vi "Smart Relay Test.vi"(8 "error in":errorcluster, 11 "IED Test in":refnum<class "IED Test.lvclass">) -> (0 "error out":errorcluster, 2 "Test Result":T1=enum."Success", 3 "IED Test out":refnum<class "IED Test.lvclass">)   [LabVIEW 2018, in "IED Test Framework.lvlib" / "IED Test.lvclass"]
uses:
  IED Test.lvclass
  C:/Program Files (x86)/National Instruments/LabVIEW 2018/vi.lib/ActorFramework/Actor/Actor.lvclass
  C:/Users/Administrator/Desktop/2018LabVIEW EMS/EMS Generic Actor/EMS Generic/EMS Generic.lvclass
  Controls/Test Result.ctl
  <vilib>/ORNL/CSEISMIC DDS/CSEISMIC DDS Base/Data Types/Controls/DeviceClass Selector.ctl
  Smart Relay Actor/Smart Relay/Smart Relay.lvclass
  C:/Users/Administrator/Desktop/2018LabVIEW EMS/IED Actors/Device DDS Communications Framework/Device DDS Communications/Device DDS Communications.lvclass
  <vilib>/ORNL/CSEISMIC DDS/CSEISMIC DDS Base/CSEISMIC DDS.lvclass/CSEISMIC DDS.ctl
  <vilib>/ORNL/CSEISMIC DDS/CSEISMIC DDS Base/Data Types/Controls/DeviceID.ctl
  <vilib>/ActorFramework/Message Enqueuer/Message Enqueuer.lvclass/Message Enqueuer.ctl
  <vilib>/ORNL/CSEISMIC DDS/CSEISMIC DDS Base/Accessors/Write DDS Reference.vi
  <vilib>/ORNL/CSEISMIC DDS/CSEISMIC DDS Base/Accessors/Read DDS Reference.vi
  <vilib>/ActorFramework/Message Enqueuer/Enqueue.vi
  <vilib>/ORNL/CSEISMIC DDS/DDS Writer/DDS Writer.lvclass
  C:/Program Files (x86)/National Instruments/LabVIEW 2018/vi.lib/ORNL/CSEISMIC DDS/CSEISMIC DDS Base/CSEISMIC DDS.lvclass
  <vilib>/ActorFramework/Stop Msg/Stop Msg.lvclass
  C:/Program Files (x86)/National Instruments/LabVIEW 2018/vi.lib/ActorFramework/Message/Message.lvclass
  <vilib>/ORNL/CSEISMIC DDS/CSEISMIC DDS Base/Error Handler.vi
  <vilib>/ActorFramework/Message Priority Queue/Priority Enqueue.vi
  <vilib>/ORNL/CSEISMIC DDS/CSEISMIC DDS Base/CSEISMIC DDS.lvclass
  Device DDS Communications Framework/Device DDS Communications/Device DDS Communications.lvclass
  <vilib>/ActorFramework/Actor/Actor.lvclass
  EMS Generic Actor/EMS Generic/EMS Generic.lvclass
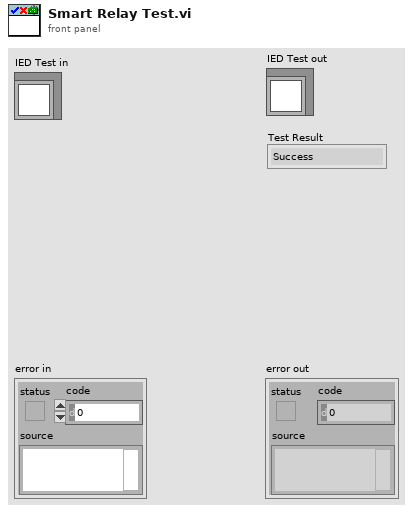
[diagram p1: front panel]
types:
  T1 = typedef "IED Test Framework.lvlib/IED Test.lvclass/Test Result.ctl" = enum16{"Invalid", "Success", "Failure", "Error", "Timeout"}
  T2 = typedef "CSEISMIC DDS.lvlib/CSEISMIC DDS.lvclass/DeviceID.ctl" = string
  T3 = typedef "CSEISMIC DDS.lvlib/CSEISMIC DDS.lvclass/DeviceClass Selector.ctl" = u16
  T4 = typedef "CSEISMIC DDS.lvlib/CSEISMIC DDS.lvclass/SmartRelay_Info.ctl" = cluster{"DeviceID":T2, "LineConfig":u8[], "NominalVoltage(V)":dbl}
  T5 = typedef "CSEISMIC DDS.lvlib/CSEISMIC DDS.lvclass/SmartRelay_Measurement.ctl" = cluster{"DeviceID":T2, "PrimaryVoltage":dbl[], "SecondaryVoltage":dbl[], "Current":dbl[], "RealPower":dbl[], "ReactivePower":dbl[], "LineConfig":u8[], "Frequency":dbl}
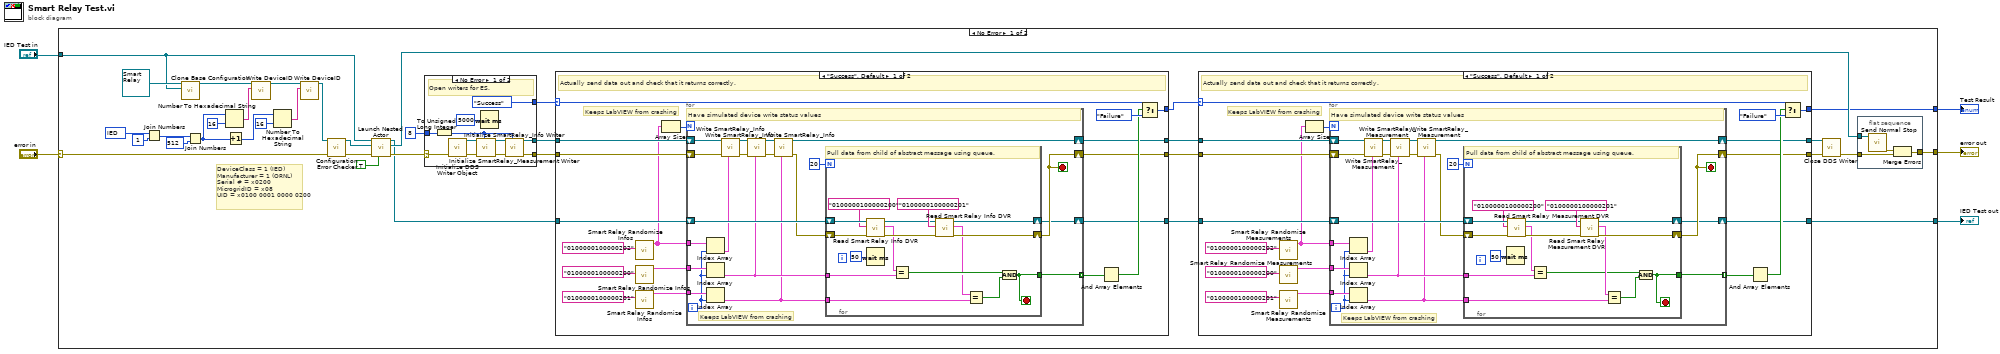
[diagram p0: block diagram]
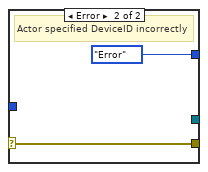
[diagram p4: hidden frame]
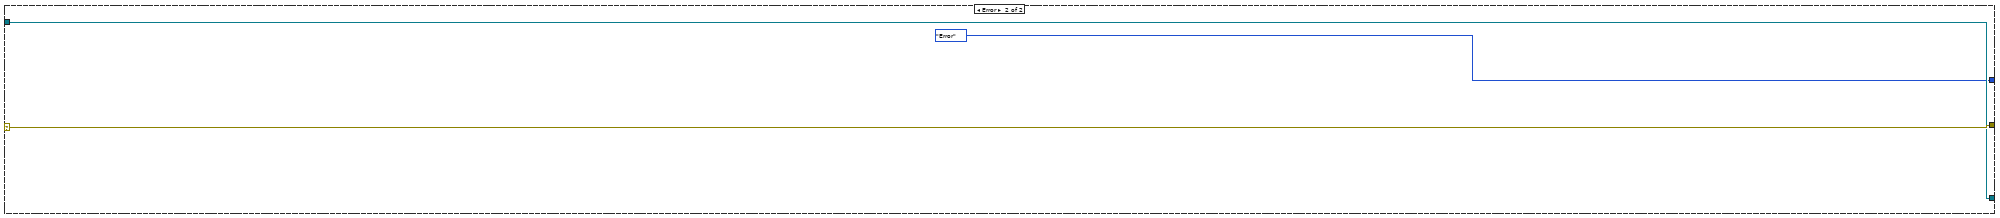
[diagram p5: hidden frame]
diagram:
  n1 = case shown="No Error" "error in" {
    selector: "error in" -> [w37 w177]
    tunnel: [w39 w177] -> w3
    tunnel: [w6 w176] -> w4
    tunnel: "IED Test in" -> [w9 w176]
    tunnel: [w13 Test_Result."Error" ("f")] -> w5
    frame No Error {
      w30 = T3 256 items=["Invalid"=0, "IED"=256, "DER"=512, "Relay"=768, "Meter"=1024, "Load"=1280, "Forecast"=1536, "Price"=1792, "Energy Storage"=513, "PV"=514, "Generator"=515, "Smart Relay"=769, "PCC"=770, "Smart Meter"=1025, "PMU"=1026, "HVAC"=1281] ("DeviceClass")
      # "DeviceClass = 1 (IED)\nManufacturer = 1 (ORNL)\nSerial # = x0200\nMicrogridID = x08\nUID = x0100 0001 0000 0200"
      n2 = Join Numbers(hi=w30, lo=u16 1 ("MicrogridID")) -> ((hi.lo)=w27:u32)
      n3 = call-dynamic "Clone Base Configuration.vi"("Source Object"=w9, "Target Object in"=refnum<class "Smart Relay.lvclass"> refnum ("Smart Relay Actor.lvlib:Smart Relay.lvclass")) -> ("Target Object out"=w10:refnum<class "Smart Relay.lvclass">)  [unwired: 9 in]
      n4 = Join Numbers(hi=w27, lo=u32 512 ("MicrogridID")) -> ((hi.lo)=w32:u64)
      n5 = Number To Hexadecimal String(1:i16 16 ("width (-)"), 2:w32) -> (0:w25:string)
      n6 = Increment(x=w32) -> (x+1=w34:u64)
      n7 = call-dynamic "Write DeviceID.vi"("DeviceID"=w25, "Device DDS Communications in"=w10) -> ("Device DDS Communications out"=w29:refnum<class "Smart Relay.lvclass">)  [unwired: 9 in]
      n8 = Number To Hexadecimal String(1:i16 16 ("width (-)"), 2:w34) -> (0:w35:string)
      n9 = call-dynamic "Write DeviceID.vi"("DeviceID"=w35, "Device DDS Communications in"=w29) -> ("Device DDS Communications out"=w12:refnum<class "Smart Relay.lvclass">)  [unwired: 9 in]
      n10 = call "Configuration Error Checker.vi"("error in"=w37, "Device DDS Communications in"=w12) -> ("error out"=w40:errorcluster, "Device DDS Communications out"=w38:refnum<class "Smart Relay.lvclass">)  [unwired: 8 in]
      n11 = call <vilib>:"Launch Nested Actor.vi"("Open Actor Core front panel? (F)"=TRUE, "error in (no error)"=w40, "Nested Actor"=w38, "Caller Actor in"=w9) -> ("error out"=w23:errorcluster, "Nested Actor's Enqueuer"=w36:refnum<class "Message Enqueuer.lvclass">, "Caller Actor out"=w7:refnum<class "IED Test.lvclass">)  [unwired: 5 in]
      n12 = case shown="No Error" w23 {
        selector: w23 -> [w170 w174]
        tunnel: [w163 w174] -> w20
        tunnel: u32 8 ("domain id") -> [w172 _]
        tunnel: [Test_Result."Success" ("Test Result in") Test_Result."Error" ("Test Result")] -> w22
        tunnel: [w162 _] -> w21
        frame No Error {
          # "Open writers for ES."
          n13 = To Unsigned Long Integer(number=w172) -> (unsigned 32bit integer=w165:u32)
          n14 = call <vilib>:"Initialize DDS Writer Object.vi"("error in"=w170) -> ("error out"=w169:errorcluster, "DDS Writer out"=w168:refnum<class "DDS Writer.lvclass">)  [unwired: 9 in]
          n15 = call <vilib>:"Initialize SmartRelay_Info Writer.vi"("MicrogridID"=w165, "error in"=w169, "DDS Writer in"=w168) -> ("error out"=w166:errorcluster, "DDS Writer out"=w167:refnum<class "DDS Writer.lvclass">)  [unwired: 7 in]
          n16 = Wait (ms)(milliseconds to wait=u32 5000) -> ()  [unwired: 1 out]
          n17 = call <vilib>:"Initialize SmartRelay_Measurement Writer.vi"("MicrogridID"=w165, "error in"=w166, "DDS Writer in"=w167) -> ("error out"=w163:errorcluster, "DDS Writer out"=w162:refnum<class "DDS Writer.lvclass">)  [unwired: 7 in]
        }
        frame Error {
          # "Actor specified DeviceID incorrectly"
        }
      }
      n18 = case shown="\"Success\", Default" w22 {
        selector: w22 -> [w120 w160]
        tunnel: w21 -> [w121 w159]
        tunnel: w7 -> [w115 w158]
        tunnel: w20 -> [w116 w161]
        tunnel: [w118 w160] -> w17
        tunnel: [w114 w161] -> w18
        tunnel: [w112 w159] -> w19
        tunnel: [w104 w158] -> w8
        frame "Success", Default {
          # "Keeps LabVIEW from crashing"
          # "Actually send data out and check that it returns correctly."
          n19 = call "Smart Relay Randomize Infos.vi"("DeviceID"=T2 "0100000100000202" ("(hi.lo)")) -> ("SmartRelay_Measurement Array out"=w111:T4[])  [unwired: 10 in]
          n20 = call "Smart Relay Randomize Infos.vi"("DeviceID"=T2 "0100000100000200" ("(hi.lo)")) -> ("SmartRelay_Measurement Array out"=w108:T4[])  [unwired: 10 in]
          n21 = call "Smart Relay Randomize Infos.vi"("DeviceID"=T2 "0100000100000201" ("(hi.lo)")) -> ("SmartRelay_Measurement Array out"=w109:T4[])  [unwired: 10 in]
          n22 = Array Size(array=w111) -> (size(s)=w113:i32)
          n23 = for {
            N: w113 -> [_]
            shift-right: [w138] -> w112
            shift-left: w121 -> [w141]
            tunnel: w111 -> [w134]
            tunnel: w109 -> [w129]
            tunnel: w108 -> [w130]
            shift-right: [w131] -> w114
            shift-left: w116 -> [w137]
            shift-right: [w123] -> w104
            shift-left: w115 -> [w133]
            tunnel: [w122] -> w105 mode=indexing
            i -> [w127]
            stop <- w131 stop-if-true
            # "Keeps LabVIEW from crashing"
            # "Have simulated device write status values"
            n24 = Index Array(array=w134, index=w127) -> (element=w126:T4)
            n25 = Index Array(array=w130, index=w127) -> (element=w125:T4)
            n26 = Index Array(array=w129, index=w127) -> (element=w124:T4)
            n27 = call <vilib>:"Write SmartRelay_Info.vi"("SmartRelay_Info"=w126, "error in"=w137, "DDS Writer in"=w141) -> ("error out"=w136:errorcluster, "DDS Writer out"=w140:refnum<class "DDS Writer.lvclass">)  [unwired: 7 in]
            n28 = call <vilib>:"Write SmartRelay_Info.vi"("SmartRelay_Info"=w125, "error in"=w136, "DDS Writer in"=w140) -> ("error out"=w135:errorcluster, "DDS Writer out"=w139:refnum<class "DDS Writer.lvclass">)  [unwired: 7 in]
            n29 = call <vilib>:"Write SmartRelay_Info.vi"("SmartRelay_Info"=w124, "error in"=w135, "DDS Writer in"=w139) -> ("error out"=w132:errorcluster, "DDS Writer out"=w138:refnum<class "DDS Writer.lvclass">)  [unwired: 7 in]
            n30 = for {
              N: 20 -> [_]
              shift-right: [w147] -> w131
              shift-left: w132 -> [w156]
              shift-right: [w148] -> w123
              shift-left: w133 -> [w157]
              tunnel: w125 -> [w151]
              tunnel: w124 -> [w149]
              tunnel: [w142] -> w122
              stop <- w142 stop-if-true
              # "Pull data from child of abstract message using queue."
              n31 = call "Read Smart Relay Info DVR.vi"("error in"=w156, "DeviceID"=T2 "0100000100000200" ("(hi.lo)"), "EMS Generic in"=w157) -> ("error out"=w153:errorcluster, "SmartRelay_Info"=w150:T4, "EMS Generic out"=w152:refnum<class "IED Test.lvclass">)  [unwired: 5 in, 1 out]
              n32 = Wait (ms)(milliseconds to wait=u32 50) -> ()  [unwired: 1 out]
              n33 = Equal?(x=w150, y=w151) -> (x = y?=w145:bool)
              n34 = call "Read Smart Relay Info DVR.vi"("error in"=w153, "DeviceID"=T2 "0100000100000201" ("(hi.lo)"), "EMS Generic in"=w152) -> ("error out"=w147:errorcluster, "SmartRelay_Info"=w143:T4, "EMS Generic out"=w148:refnum<class "IED Test.lvclass">)  [unwired: 5 in, 1 out]
              n35 = Equal?(x=w143, y=w149) -> (x = y?=w144:bool)
              n36 = And(x=w145, y=w144) -> (x .and. y?=w142:bool)
            }
          }
          n37 = And Array Elements(Boolean array=w105) -> (logical AND=w117:bool)
          n38 = Select(t=w120, s=w117, f=Test_Result."Failure") -> (s? t:f=w118:T1)
        }
        frame "Error" {
        }
      }
      n39 = case shown="\"Success\", Default" w17 {
        selector: w17 -> [w62 w102]
        tunnel: w19 -> [w63 w101]
        tunnel: w8 -> [w57 w100]
        tunnel: w18 -> [w58 w103]
        tunnel: [w60 w102] -> w13
        tunnel: [w56 w103] -> w15
        tunnel: [w54 w101] -> w16
        tunnel: [w47 w100] -> w6
        frame "Success", Default {
          # "Keeps LabVIEW from crashing"
          # "Actually send data out and check that it returns correctly."
          n40 = call "Smart Relay Randomize Measurements.vi"("DeviceID"=T2 "0100000100000202" ("(hi.lo)")) -> ("SmartRelay_Measurement Array out"=w53:T5[])  [unwired: 10 in]
          n41 = call "Smart Relay Randomize Measurements.vi"("DeviceID"=T2 "0100000100000200" ("(hi.lo)")) -> ("SmartRelay_Measurement Array out"=w48:T5[])  [unwired: 10 in]
          n42 = call "Smart Relay Randomize Measurements.vi"("DeviceID"=T2 "0100000100000201" ("(hi.lo)")) -> ("SmartRelay_Measurement Array out"=w49:T5[])  [unwired: 10 in]
          n43 = Array Size(array=w53) -> (size(s)=w55:i32)
          n44 = for {
            N: w55 -> [_]
            shift-right: [w80] -> w54
            shift-left: w63 -> [w83]
            tunnel: w53 -> [w76]
            tunnel: w49 -> [w71]
            tunnel: w48 -> [w72]
            shift-right: [w73] -> w56
            shift-left: w58 -> [w79]
            shift-right: [w67] -> w47
            shift-left: w57 -> [w75]
            tunnel: [w64] -> w46 mode=indexing
            i -> [w69]
            stop <- w73 stop-if-true
            # "Keeps LabVIEW from crashing"
            # "Have simulated device write status values"
            n45 = Index Array(array=w76, index=w69) -> (element=w68:T5)
            n46 = Index Array(array=w72, index=w69) -> (element=w66:T5)
            n47 = Index Array(array=w71, index=w69) -> (element=w65:T5)
            n48 = call <vilib>:"Write SmartRelay_Measurement.vi"("SmartRelay_Measurement"=w68, "error in"=w79, "DDS Writer in"=w83) -> ("error out"=w78:errorcluster, "DDS Writer out"=w82:refnum<class "DDS Writer.lvclass">)  [unwired: 7 in]
            n49 = call <vilib>:"Write SmartRelay_Measurement.vi"("SmartRelay_Measurement"=w66, "error in"=w78, "DDS Writer in"=w82) -> ("error out"=w77:errorcluster, "DDS Writer out"=w81:refnum<class "DDS Writer.lvclass">)  [unwired: 7 in]
            n50 = call <vilib>:"Write SmartRelay_Measurement.vi"("SmartRelay_Measurement"=w65, "error in"=w77, "DDS Writer in"=w81) -> ("error out"=w74:errorcluster, "DDS Writer out"=w80:refnum<class "DDS Writer.lvclass">)  [unwired: 7 in]
            n51 = for {
              N: 20 -> [_]
              shift-right: [w93] -> w73
              shift-left: w74 -> [w98]
              shift-right: [w92] -> w67
              shift-left: w75 -> [w99]
              tunnel: w66 -> [w91]
              tunnel: w65 -> [w90]
              tunnel: [w85] -> w64
              stop <- w85 stop-if-true
              # "Pull data from child of abstract message using queue."
              n52 = Wait (ms)(milliseconds to wait=u32 50) -> ()  [unwired: 1 out]
              n53 = call "Read Smart Relay Measurement DVR.vi"("error in"=w98, "DeviceID"=T2 "0100000100000200" ("(hi.lo)"), "EMS Generic in"=w99) -> ("error out"=w94:errorcluster, "SmartRelay_Measurement"=w89:T5, "EMS Generic out"=w95:refnum<class "IED Test.lvclass">)  [unwired: 5 in, 1 out]
              n54 = Equal?(x=w89, y=w91) -> (x = y?=w87:bool)
              n55 = call "Read Smart Relay Measurement DVR.vi"("error in"=w94, "DeviceID"=T2 "0100000100000201" ("(hi.lo)"), "EMS Generic in"=w95) -> ("error out"=w93:errorcluster, "SmartRelay_Measurement"=w88:T5, "EMS Generic out"=w92:refnum<class "IED Test.lvclass">)  [unwired: 5 in, 1 out]
              n56 = Equal?(x=w88, y=w90) -> (x = y?=w86:bool)
              n57 = And(x=w87, y=w86) -> (x .and. y?=w85:bool)
            }
          }
          n58 = And Array Elements(Boolean array=w46) -> (logical AND=w59:bool)
          n59 = Select(t=w62, s=w59, f=Test_Result."Failure") -> (s? t:f=w60:T1)
        }
        frame "Error" {
        }
      }
      n60 = call <vilib>:"Close DDS Writer.vi"("error in"=w15, "DDS Writer in"=w16) -> ("error out"=w14:errorcluster)  [unwired: 9 in]
      n61 = flat-sequence {
        tunnel: w36 -> [w45]
        tunnel: [w43] -> w39
        tunnel: w14 -> [w42]
        frame #0 {
          n62 = call <vilib>:"Send Normal Stop.vi"("Message Enqueuer"=w45) -> ("error out"=w44:errorcluster)  [unwired: 10 in]
          n63 = Merge Errors(w44, w42) -> (w43:errorcluster)
        }
      }
    }
    frame Error {
    }
  }
  "error out" <- w3
  "IED Test out" <- w4
  "Test Result" <- w5
